vi "MeasureToBuffer.vi"(7 "SMU":T2, 8 "Error In":errorcluster, 9 "Buffer":u8=1 min=1 max=2 step=1, 10 "Measure Function":T1, 11 "Keithley 2602 In":refnum<visa-resource-name>) -> (0 "Error Out":errorcluster, 2 "Last Reading":dbl, 3 "Keithley 2602 Out":refnum<visa-resource-name>)   [LabVIEW 2012, in "Keithley-2602.lvlib"]
uses:
  Keithley-2602.lvlib
  Controls/SMU.ctl
  Controls/MeasureFunction.ctl
panel:
  out "Command":string
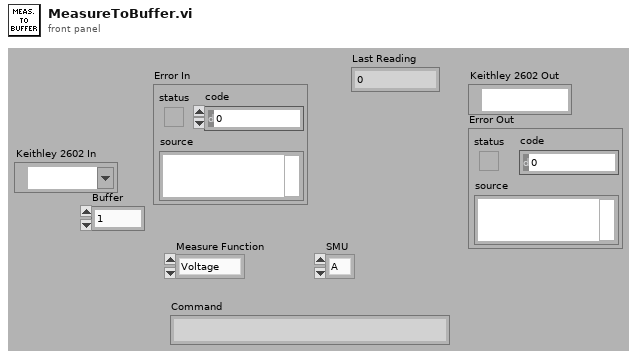
[diagram p1: front panel]
types:
  T1 = typedef "Keithley-2602.lvlib/MeasureFunction.ctl" = enum16{"Voltage", "Current", "Resistance", "Power"}
  T2 = typedef "Keithley-2602.lvlib/SMU.ctl" = enum16{"A", "B"}
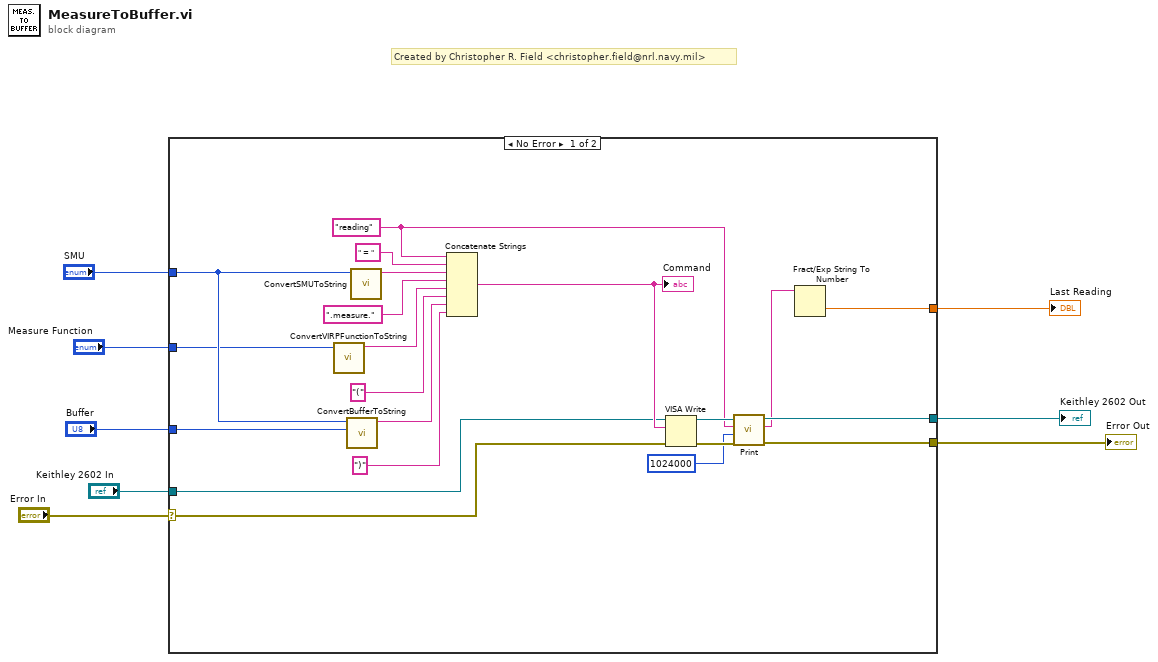
[diagram p0: block diagram]
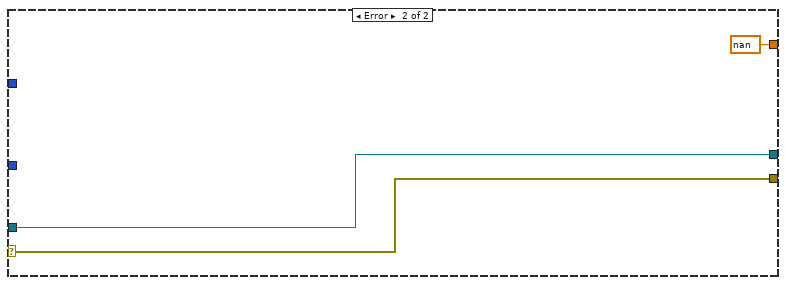
[diagram p2: hidden frame]
diagram:
  # "Created by Christopher R. Field <christopher.field@nrl.navy.mil>"
  n1 = case shown="No Error" "Error In" {
    selector: "Error In" -> [w9 w31]
    tunnel: "Buffer" -> [w24 _]
    tunnel: [w19 w32] -> w7
    tunnel: [w18 w31] -> w6
    tunnel: [w16 nan] -> w5
    tunnel: "SMU" -> [w12 _]
    tunnel: "Measure Function" -> [w11 _]
    tunnel: "Keithley 2602 In" -> [w10 w32]
    frame No Error {
      w13 = "reading"
      n2 = call "ConvertVIRPFunctionToString.vi"("Function"=w11) -> ("Function"=w27:string)  [unwired: 10 in]
      n3 = call "ConvertBufferToString.vi"("Buffer"=w24, "SMU"=w12) -> ("Buffer"=w23:string)  [unwired: 9 in]
      n4 = call "ConvertSMUToString.vi"("SMU"=w12) -> ("Channel"=w29:string)  [unwired: 10 in]
      n5 = Concatenate Strings(w13, " = ", w29, ".measure.", w27, "(" ("string"), w23, ")" ("string")) -> (w25:string)
      "Command" <- w25
      n6 = VISA Write(VISA resource name=w10, write buffer=w25, error in (no error)=w9) -> (VISA resource name out=w21:refnum<visa-resource-name>, error out=w20:errorcluster)  [unwired: 1 out]
      n7 = call "Print.vi"("Error In"=w20, "Byte Count"=u32 1024000 ("byte count"), "Attribute"=w13, "Kiethley 2602 In"=w21) -> ("Error Out"=w18:errorcluster, "Output"=w17:string, "Keithley 2602 Out"=w19:refnum<visa-resource-name>)  [unwired: 5 in]
      n8 = Fract/Exp String To Number(string=w17) -> (number=w16:dbl)  [unwired: 3 in, 1 out]
    }
    frame Error {
    }
  }
  "Keithley 2602 Out" <- w7
  "Error Out" <- w6
  "Last Reading" <- w5
